vi "多参校准第一步.vi"() -> (1 "校准模式选择":enum32{"单点校准", "多点校准"}(ring), 2 "校准探头":u16, 3 "继续执行":bool)   [LabVIEW 2016, in "斯坦道仪器.lvlib"]
panel:
  in  "取消":bool
  in  "下一步":bool
  in  "校准模式":enum32{"单点校准", "多点校准"}(radio)
  in  "校准区探头选择":u16(ring)=10 items=["氨氮"=3, "pH值"=10, "溶解氧"=11, "电导率"=12, "浊度"=13, "叶绿素a"=14, "藻密度"=15, "蓝绿藻"=16, "氧化还原电位"=17, "溶解氧%"=18, "盐度"=19]
  # "请选择校准参数："
  # "请选择校准模式："
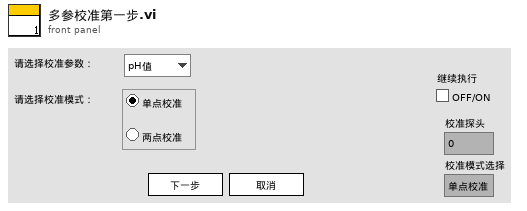
[diagram p1: front panel]
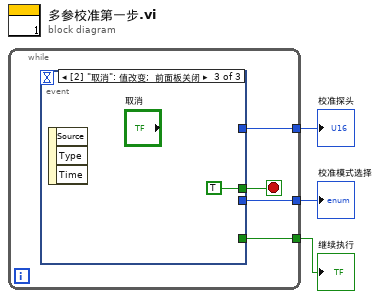
[diagram p0: block diagram]
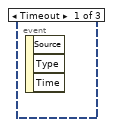
[diagram p2: hidden frame]
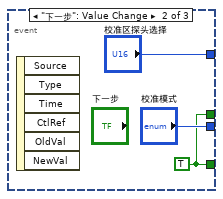
[diagram p3: hidden frame]
diagram:
  n1 = while {
    tunnel: [w7] -> w2
    tunnel: [w6] -> w1
    tunnel: [w5] -> w3
    stop <- w4 stop-if-true
    n2 = event shown="[2] \"取消\": 值改变;  前面板关闭" {
      selector: _ -> [_ _ _]
      dyn-events: _ -> [_ _ _]
      timeout: _ -> [_ _ _]
      tunnel: [_ "校准区探头选择" _] -> w7
      tunnel: [_ "校准模式" _] -> w6
      tunnel: [_ w8 _] -> w5
      tunnel: [_ w8 TRUE ("继续执行")] -> w4
      event Timeout {
        n3 = event-data() -> ()  [unwired: 1 in, 3 out]
      }
      event "下一步": Value Change {
        w8 = TRUE ("继续执行")
        n4 = event-data() -> ()  [unwired: 1 in, 6 out]
      }
      event "取消": Value Change; Panel Close {
        n5 = event-data() -> ()  [unwired: 1 in, 3 out]
      }
    }
  }
  "继续执行" <- w3
  "校准探头" <- w2
  "校准模式选择" <- w1
